vi "completeCycle.vi"(8 "error in (no error)":errorcluster, 11 "Model in":refnum<class "Model.lvclass">) -> (0 "error out":errorcluster, 2 "preconditiongCompleteIsTrue":bool, 3 "Model out":refnum<class "Model.lvclass">)   [LabVIEW 2015, in "Model.lvclass"]
uses:
  Model.lvclass
  Model.lvclass/Model.ctl
  UserEvents/UserEvents.lvclass/UserEvents.ctl
  ApplicationElements/PreconditioningMonitor/PreconditioningMonitor.lvclass
  UserEvents/UserEvents.lvclass
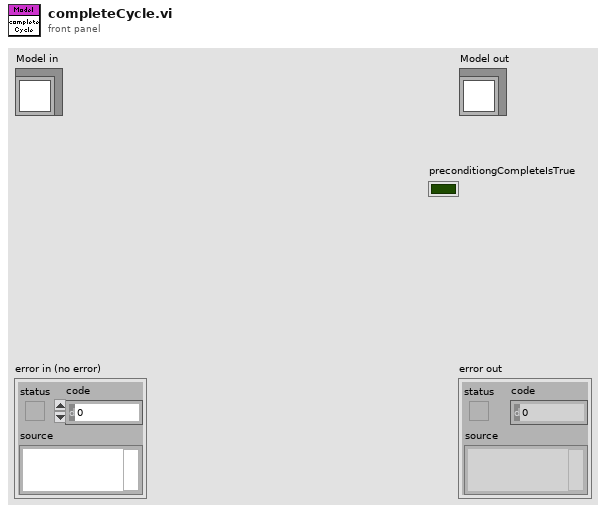
[diagram p1: front panel]
types:
  T1 = typedef "M1M3SSSTypedefs.lvlib/PubDataEvents.ctl" = cluster{"State":refnum<user-event>, "ErrorCode":refnum<user-event>, "OutputData":refnum<user-event>, "InputData":refnum<user-event>, "ControllerData":refnum<user-event>, "TestStatus":refnum<user-event>, "LogPath":refnum<user-event>, "StiffnessData":refnum<user-event>, "PreconditioningCycle":refnum<user-event>}
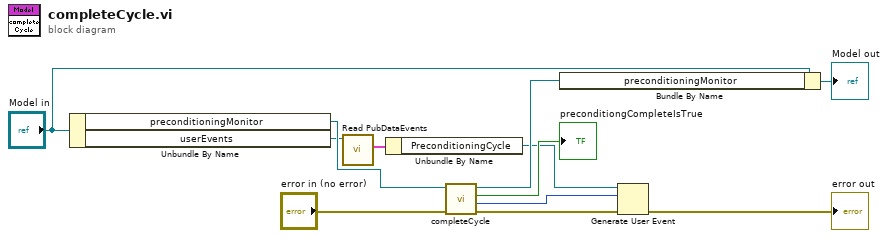
[diagram p0: block diagram]
diagram:
  n1 = Unbundle By Name("Model in") -> ("preconditioningMonitor"=w12:refnum<class "PreconditioningMonitor.lvclass">, "userEvents"=w7:refnum<class "UserEvents.lvclass">)
  n2 = call "Read PubDataEvents.vi"("UserEvents in"=w7) -> ("PubDataEvents"=w6:T1)  [unwired: 9 in, 1 out]
  n3 = Unbundle By Name(w6) -> ("PreconditioningCycle"=w4:refnum<user-event>)
  n4 = call "completeCycle.vi"("error in (no error)"="error in (no error)", "PreconditioningMonitor in"=w12) -> ("error out"=w2:errorcluster, "preconditioningCycle"=w3:u32, "preconditiongCompleteIsTrue"=→"preconditiongCompleteIsTrue":bool, "PreconditioningMonitor out"=w9:refnum<class "PreconditioningMonitor.lvclass">)  [unwired: 6 in]
  n5 = Bundle By Name(cluster="Model in", "preconditioningMonitor"=w9) -> (→"Model out":refnum<class "Model.lvclass">)
  n6 = Generate User Event(user event=w4, event data cluster=w3, error in=w2) -> (error out=→"error out":errorcluster)  [unwired: 1 in, 1 out]
